vi "ACT_LabView3_Task3_Team072.vi"() -> ()   [LabVIEW 2016]
panel:
  out "Heads":dbl
  out "Tails":dbl
  in  "# of Coin Flips":dbl
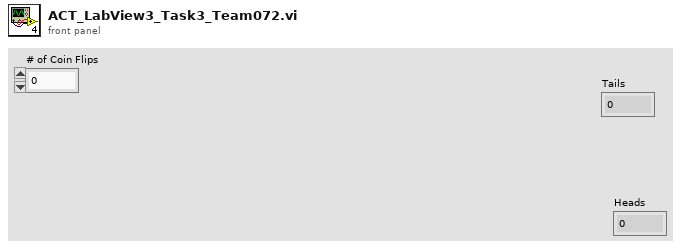
[diagram p1: front panel]
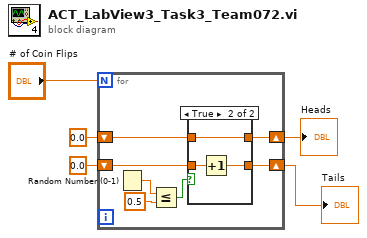
[diagram p0: block diagram]
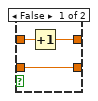
[diagram p2: hidden frame]
diagram:
  n1 = for {
    N: "# of Coin Flips" -> [_]
    shift-right: [w12] -> w4
    shift-left: 0.0 -> [w10]
    shift-right: [w11] -> w3
    shift-left: 0.0 -> [w9]
    n2 = Random Number (0-1)() -> (number: 0 to 1=w7:dbl)
    n3 = Less Or Equal?(x=w7, y=0.5) -> (x <= y?=w6:bool)
    n4 = case shown="True" w6 {
      tunnel: w10 -> [w13 w18]
      tunnel: [w13 w17] -> w12
      tunnel: [w15 w16] -> w11
      tunnel: w9 -> [w14 w16]
      frame False {
        n5 = Increment(x=w14) -> (x+1=w15:dbl)
      }
      frame True {
        n6 = Increment(x=w18) -> (x+1=w17:dbl)
      }
    }
  }
  "Heads" <- w3
  "Tails" <- w4
